vi "Msg Send Priority Queue Message.vi"(5 "timeout in ms (-1)":i32=-1, 6 "error in (no error)":errorcluster, 7 "Data":variant, 8 "Message":string, 9 "queue":refnum<queue>) -> (0 "error out":errorcluster, 1 "timed out?":bool, 3 "queue out":refnum<queue>)   [LabVIEW 2014]
doc: "Sends a high priority message to the front specified message queue (or event structure). This function awaits a response from the recipient which should be sent with Msg Send Response.vi.\n\nThis is part of the Msg suite, intended to make messaging architectures in LabVIEW\nSee the template \"Message Based Application Template.vi\" for normal usage.\n\nCopyright 2005-2016 Jason Sommerville\n\nSends a response to the original sender of a message (sent via Msg Send Message). It should form bookends with Msg Get Message in the message handling loop.\n\nThis is part of the Msg suite, intended to make messaging architectures in LabVIEW\nSee the template \"Message Based Application Template.vi\" for normal usage.\n\nCopyright 2005-2016 Jason Sommerville\n\nThis VI may be freely used, modified or distributed under the BSD license."
uses:
  Message Cluster.ctl
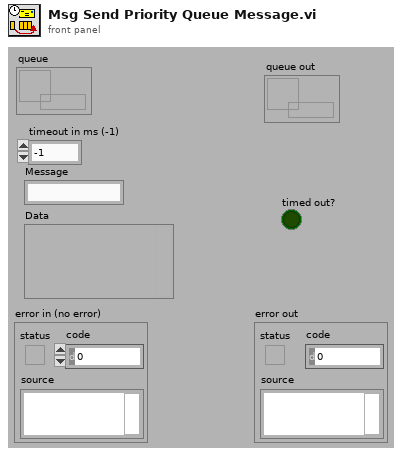
[diagram p1: front panel]
types:
  T1 = cluster{"Message":string, "Data":variant, refnum<k0>}
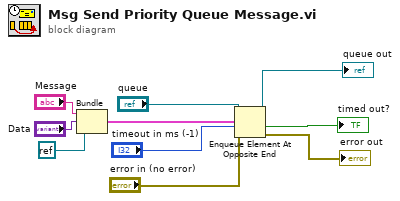
[diagram p0: block diagram]
diagram:
  n1 = Bundle("Message"="Message", "Data"="Data", refnum<k0> refnum) -> (w3:T1)  [unwired: 1 in]
  n2 = Enqueue Element At Opposite End(queue="queue", element=w3, timeout in ms (-1)="timeout in ms (-1)", error in (no error)="error in (no error)") -> (queue out=→"queue out":refnum<queue>, timed out?=→"timed out?":bool, error out=→"error out":errorcluster)
